vi "Owning Node.vi"(8 "error in (no error)":errorcluster, 11 "Group in":refnum<class "Group.lvclass">) -> (0 "error out":errorcluster, 2 "Owning Node":string, 3 "Group out":refnum<class "Group.lvclass">)   [LabVIEW 2020, in "VolatusConfig.lvlib" / "Group.lvclass"]
uses:
  Group.lvclass
  C:/dev/lv20CE/relink/lv-volatus/VolatusConfig/VolatusConfigElement/VolatusConfigElement.lvclass
  Meta Type.ctl
  VolatusConfigElement/VolatusConfigElement.lvclass/VolatusConfigElement.ctl
  VolatusConfigElement/Element.vi
  lv-cdm/CDM-Config/Config Lookup/Match Meta.vi
  lv-cdm/CDM-Config/Config Element/Owner.vi
  lv-cdm/CDM-Config/Config Filter/Config Lookup.lvclass
  VolatusConfig.lvlib
  lv-cdm/CDM-Config/Config Element/Config Element.lvclass
  VolatusConfigElement/VolatusConfigElement.lvclass
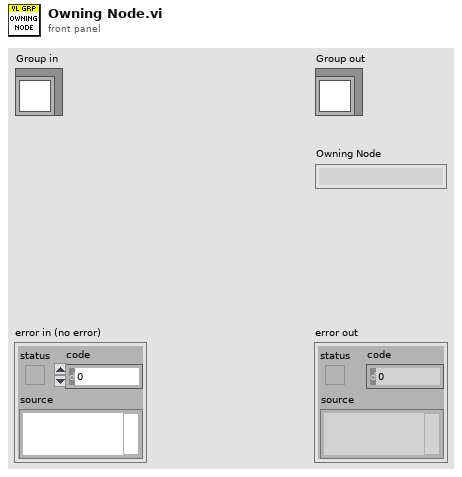
[diagram p1: front panel]
types:
  T1 = typedef "VolatusConfig.lvlib/Meta Type.ctl" = enum16{"UNKNOWN", "VL_System", "VL_Cluster", "VL_Node", "VL_Task", "VL_Group", "VL_Channel", "VL_Task_List", "VL_Scaling", "VL_Sensor", "VL_Sensor_List", "VL_Scale"}
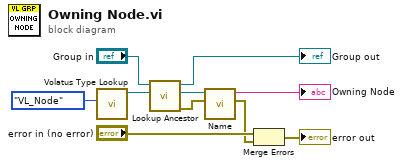
[diagram p0: block diagram]
diagram:
  n1 = call "Volatus Type Lookup.vi"("Meta Type"=Meta_Type."VL_Node") -> ("Config Lookup out"=w8:refnum<class "Config Lookup.lvclass">)  [unwired: 9 in, 1 out]
  n2 = call "Lookup Ancestor.vi"("Lookup"=w8, "VolatusConfigElement in"="Group in") -> ("error out"=w4:errorcluster, "Ancestor"=w7:refnum<class "Config Element.lvclass">, "VolatusConfigElement out"=→"Group out":refnum<class "Group.lvclass">)  [unwired: 7 in]
  n3 = call "Name.vi"("error in (no error)"=w4, "Config Element in"=w7) -> ("error out"=w3:errorcluster, "Name"=→"Owning Node":string)  [unwired: 8 in]
  n4 = Merge Errors("error in (no error)", w3) -> (→"error out":errorcluster)
